vi "Chart Buffer.vi"(0 "Wfm In":sgl[][](array[numeric]), 1 "Reset?":bool, 5 "Chart History":i32=500) -> (6 "Wfm Out":sgl[][](array[numeric]))   [LabVIEW 2012, in "Preview Window.lvlib" / "Preview.lvclass"]
uses:
  Preview.lvclass
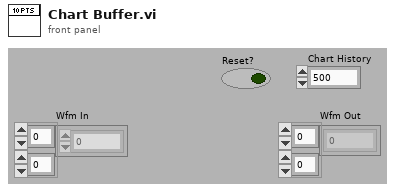
[diagram p1: front panel]
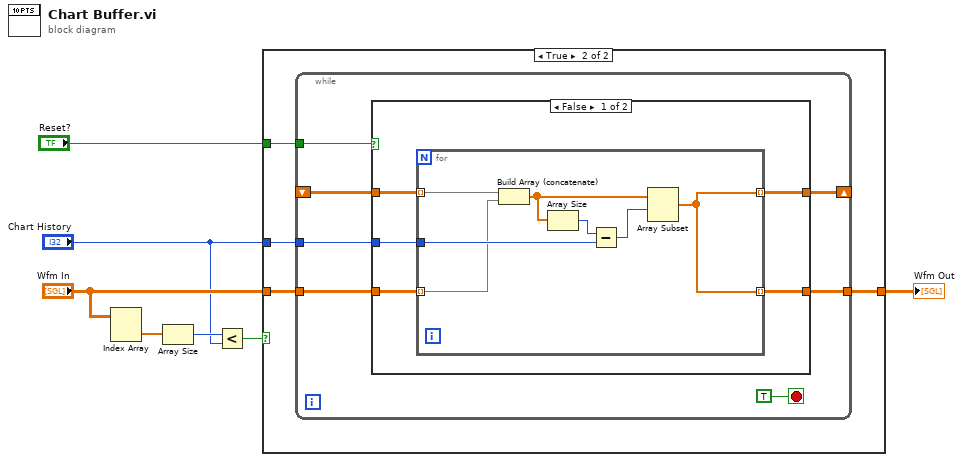
[diagram p0: block diagram]
diagram:
  n1 = Index Array(array="Wfm In") -> (element=w1:sgl[])  [unwired: 2 in]
  n2 = Array Size(array=w1) -> (size(s)=w4:i32)
  n3 = Less?(x=w4, y="Chart History") -> (x < y?=w5:bool)
  n4 = case shown="True" w5 {
    tunnel: [w8 w11] -> w7
    tunnel: "Wfm In" -> [w8 w12]
    tunnel: "Chart History" -> [_ w10]
    tunnel: "Reset?" -> [_ w9]
    frame False {
    }
    frame True {
      n5 = while {
        tunnel: w12 -> [w18]
        shift-right: [w17] -> _
        shift-left: _ -> [w15]
        tunnel: [w16] -> w11
        tunnel: w10 -> [w14]
        tunnel: w9 -> [w13]
        stop <- TRUE stop-if-true
        n6 = case shown="False" w13 {
          tunnel: w18 -> [w23 w32]
          tunnel: [w21 w32] -> w17
          tunnel: [w20 w32] -> w16
          tunnel: w15 -> [w24 _]
          tunnel: w14 -> [w22 _]
          frame False {
            n7 = for {
              tunnel: w23 -> [w26] mode=indexing
              tunnel: w24 -> [w31] mode=indexing
              tunnel: w22 -> [w28]
              tunnel: [w25] -> w21 mode=indexing
              tunnel: [w25] -> w20 mode=indexing
              n8 = Build Array (concatenate)(w31, w26) -> (w30:sgl[])
              n9 = Array Size(array=w30) -> (size(s)=w29:i32)
              n10 = Subtract(x=w29, y=w28) -> (x-y=w27:i32)
              n11 = Array Subset(array=w30, index=w27) -> (w25:sgl[])  [unwired: 1 in]
            }
          }
          frame True {
          }
        }
      }
    }
  }
  "Wfm Out" <- w7
